vi "Clear Table.vi"(8 "error in (no error)":errorcluster caption="错误输入（无错误）", 11 "DataTable 输入":refnum<class "DataTable.lvclass"> caption="DNL_LabVIEW Object in") -> (0 "error out":errorcluster caption="错误输出", 3 "DataTable 输出":refnum<class "DataTable.lvclass"> caption="DNL_LabVIEW Object out")   [LabVIEW 2012, in "Data Grid VIEW.lvlib" / "DataTable.lvclass"]
uses:
  DataTable.lvclass
  DataTable.lvclass/DataTable.ctl
  System.Data
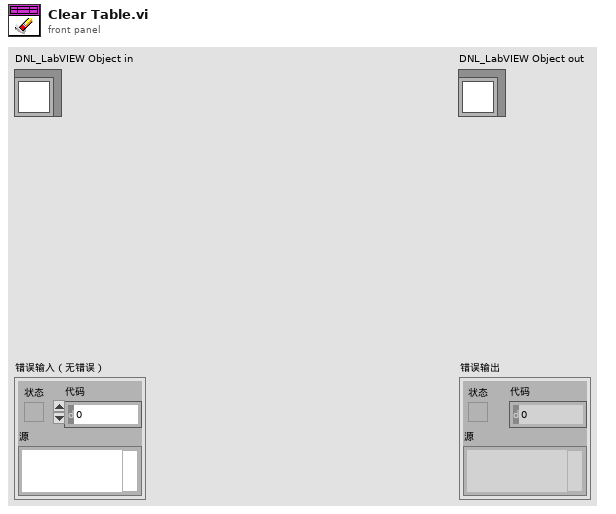
[diagram p1: front panel]
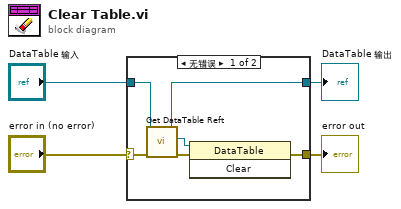
[diagram p0: block diagram]
diagram:
  n1 = case shown="无错误" "error in (no error)" {
    selector: "error in (no error)" -> [w7 w12]
    tunnel: [w5 w12] -> w3
    tunnel: [w8 w11] -> w1
    tunnel: "DataTable 输入" -> [w10 w11]
    frame No Error {
      n2 = call "Get DataTable Reft.vi"("error in (no error)"=w7, "DataTable输入"=w10) -> ("error out"=w6:errorcluster, "DataTable"=w9:refnum<k24>, "DataTable输出"=w8:refnum<class "DataTable.lvclass">)  [unwired: 7 in]
      n3 = invoke class="DataTable" method="Clear"(reference=w9, error in=w6) -> (error out=w5:errorcluster)  [unwired: 1 in, 2 out]
    }
    frame Error {
    }
  }
  "error out" <- w3
  "DataTable 输出" <- w1
